vi "Get_ADAM_Ch_names_server.vi"(1 "Channel names set":T1) -> (0 "Ch names":string[](array[string]))   [LabVIEW 2022 SP3]
uses:
  ADAM Client/Sub VIs/ADAM Controls/Channel_names.ctl
  ADAM Client/Sub VIs/ADAM Controls/Channel_State.ctl
  Sub VI's/Channel_Description_Global.vi
  ADAM_Global.vi
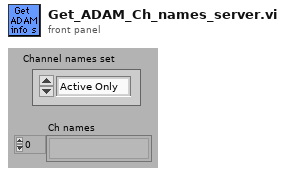
[diagram p1: front panel]
types:
  T1 = typedef "Channel_names.ctl" = enum16{"Active Only", "Active + Off", "All Channels", "Changeable Only", "Always Off", "Always On", "Always Off or On"}
  T2 = typedef "Ch_description_ADAM.ctl" = cluster{"Ch Name":string, "Type":T3, "Function":T4, "Ch State":T5, "Calibration type":T6, "A":dbl, "B":dbl, "C":dbl, "D":dbl, "Comments":string, "Address":T7, "String":string, "Duty":u16}
  T3 = typedef "Module_type_ADAM.ctl" = string
  T4 = typedef "Function_ADAM.ctl" = enum16{"Analogue Input", "Digital Input", "Event counter", "Event rate", "Analogue Output", "Digital Output", "Relay Output"}
  T5 = typedef "Channel_State.ctl" = enum16{"On", "Off", "Always On", "Always Off"}
  T6 = typedef "Calib_type_ADAM.ctl" = string
  T7 = typedef "Address.ctl" = cluster{"Main":i32, "Ch.":i32, "Sub":i32, "Port Name":string}
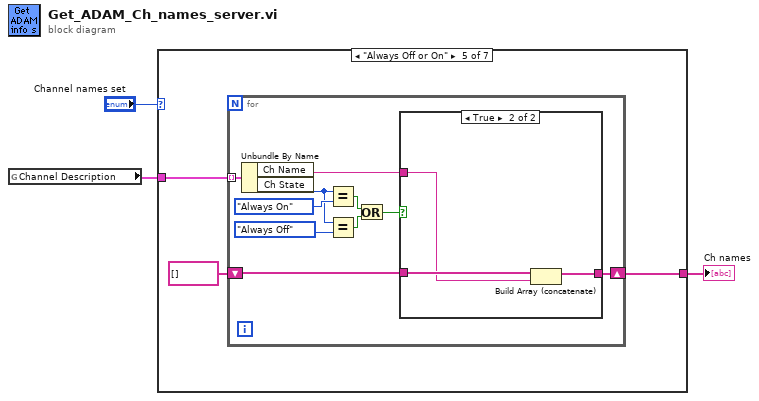
[diagram p0: block diagram]
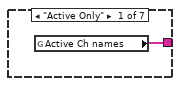
[diagram p2: hidden frame]
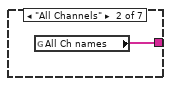
[diagram p3: hidden frame]
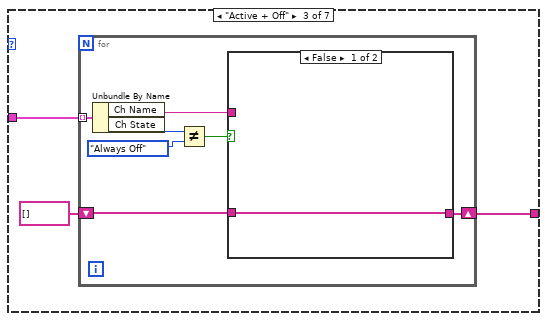
[diagram p4: hidden frame]
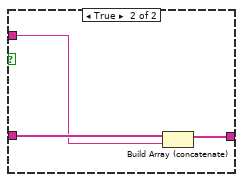
[diagram p5: hidden frame]
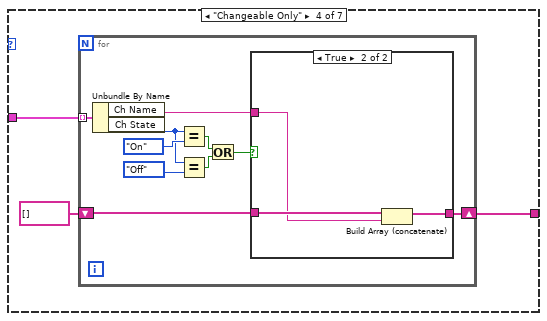
[diagram p6: hidden frame]
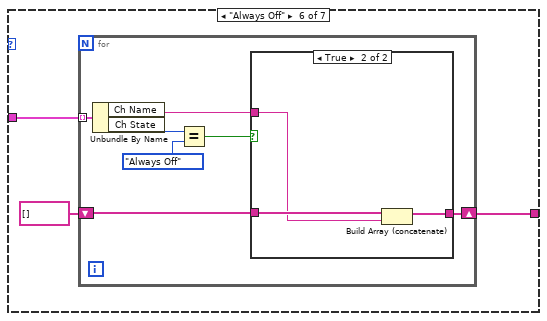
[diagram p9: hidden frame]
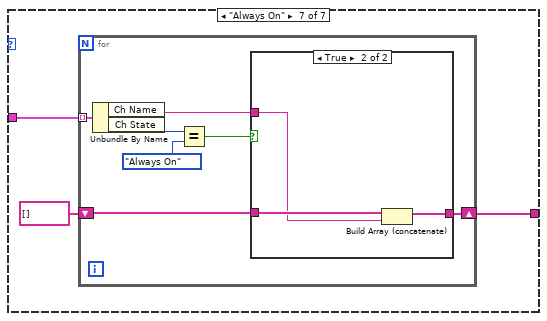
[diagram p11: hidden frame]
diagram:
  n1 = global read "Channel_Description_Global.vi" "Channel Description"() -> (w1:T2[])
  n2 = case shown="\"Always Off or On\"" "Channel names set" {
    tunnel: [w4 w5 w7 w21 w38 w55 w69] -> w2
    tunnel: w1 -> [_ _ w6 w20 w37 w54 w68]
    frame "Active Only" {
      n3 = global read "ADAM_Global.vi" "Active Ch names"() -> (w4:string[])
    }
    frame "All Channels" {
      n4 = global read "ADAM_Global.vi" "All Ch names"() -> (w5:string[])
    }
    frame "Active + Off" {
      n5 = for {
        tunnel: w6 -> [w15] mode=indexing
        shift-right: [w10] -> w7
        shift-left: string[] [] -> [w11]
        n6 = Unbundle By Name(w15) -> ("Ch Name"=w9:string, "Ch State"=w14:T5)
        n7 = Not Equal?(x=w14, y=Channel_State."Always Off" ("Channel State")) -> (x != y?=w12:bool)
        n8 = case shown="False" w12 {
          tunnel: w11 -> [w16 w19]
          tunnel: [w16 w18] -> w10
          tunnel: w9 -> [_ w17]
          frame False {
          }
          frame True {
            n9 = Build Array (concatenate)(w19, w17) -> (w18:string[])
          }
        }
      }
    }
    frame "Changeable Only" {
      n10 = for {
        tunnel: w20 -> [w32] mode=indexing
        shift-right: [w29] -> w21
        shift-left: string[] [] -> [w30]
        n11 = Unbundle By Name(w32) -> ("Ch Name"=w28:string, "Ch State"=w25:T5)
        n12 = Equal?(x=w25, y=Channel_State."On" ("Channel State")) -> (x = y?=w27:bool)
        n13 = Equal?(x=w25, y=Channel_State."Off" ("Channel State")) -> (x = y?=w23:bool)
        n14 = Or(x=w27, y=w23) -> (x .or. y?=w24:bool)
        n15 = case shown="True" w24 {
          tunnel: w30 -> [w33 w36]
          tunnel: [w33 w35] -> w29
          tunnel: w28 -> [_ w34]
          frame False {
          }
          frame True {
            n16 = Build Array (concatenate)(w36, w34) -> (w35:string[])
          }
        }
      }
    }
    frame "Always Off or On" {
      n17 = for {
        tunnel: w37 -> [w49] mode=indexing
        shift-right: [w46] -> w38
        shift-left: string[] [] -> [w47]
        n18 = Unbundle By Name(w49) -> ("Ch Name"=w45:string, "Ch State"=w42:T5)
        n19 = Equal?(x=w42, y=Channel_State."Always On" ("Channel State")) -> (x = y?=w44:bool)
        n20 = Equal?(x=w42, y=Channel_State."Always Off" ("Channel State")) -> (x = y?=w40:bool)
        n21 = Or(x=w44, y=w40) -> (x .or. y?=w41:bool)
        n22 = case shown="True" w41 {
          tunnel: w47 -> [w50 w53]
          tunnel: [w50 w52] -> w46
          tunnel: w45 -> [_ w51]
          frame False {
          }
          frame True {
            n23 = Build Array (concatenate)(w53, w51) -> (w52:string[])
          }
        }
      }
    }
    frame "Always Off" {
      n24 = for {
        tunnel: w54 -> [w63] mode=indexing
        shift-right: [w60] -> w55
        shift-left: string[] [] -> [w61]
        n25 = Unbundle By Name(w63) -> ("Ch Name"=w59:string, "Ch State"=w58:T5)
        n26 = Equal?(x=w58, y=Channel_State."Always Off" ("Channel State")) -> (x = y?=w57:bool)
        n27 = case shown="True" w57 {
          tunnel: w61 -> [w64 w67]
          tunnel: [w64 w66] -> w60
          tunnel: w59 -> [_ w65]
          frame False {
          }
          frame True {
            n28 = Build Array (concatenate)(w67, w65) -> (w66:string[])
          }
        }
      }
    }
    frame "Always On" {
      n29 = for {
        tunnel: w68 -> [w77] mode=indexing
        shift-right: [w74] -> w69
        shift-left: string[] [] -> [w75]
        n30 = Unbundle By Name(w77) -> ("Ch Name"=w73:string, "Ch State"=w72:T5)
        n31 = Equal?(x=w72, y=Channel_State."Always On" ("Channel State")) -> (x = y?=w71:bool)
        n32 = case shown="True" w71 {
          tunnel: w75 -> [w78 w81]
          tunnel: [w78 w80] -> w74
          tunnel: w73 -> [_ w79]
          frame False {
          }
          frame True {
            n33 = Build Array (concatenate)(w81, w79) -> (w80:string[])
          }
        }
      }
    }
  }
  "Ch names" <- w2
